vi "find_nearest.vi"(0 "Array":dbl[](array[numeric]), 9 "element":dbl, 11 "start index":i32) -> (4 "nearest element":dbl, 15 "min index(es)":i32)   [LabVIEW 2023]
doc: "Used find the nearest element to given number in an array."
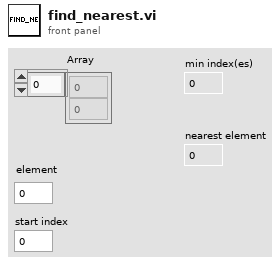
[diagram p1: front panel]
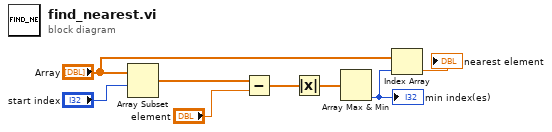
[diagram p0: block diagram]
diagram:
  n1 = Array Subset(array="Array", index="start index") -> (w5:dbl[])  [unwired: 1 in]
  n2 = Subtract(x=w5, y="element") -> (x-y=w8:dbl[])
  n3 = Absolute Value(x=w8) -> (abs(x)=w7:dbl[])
  n4 = Array Max & Min(array=w7) -> (min index (indices)=w2:i32)  [unwired: 3 out]
  "min index(es)" <- w2
  n5 = Index Array(array="Array", index=w2) -> (element=→"nearest element":dbl)
